vi "Get Command Line Arguments.vi"(8 "error in (no error)":errorcluster) -> (0 "error out":errorcluster, 2 "arguments":string[](array[string]), 3 "application name":string)   [LabVIEW 2020]
doc: "Returns the arguments passed from the command line when LabVIEW or a LabVIEW-built application launched. User-defined arguments start after two hyphens (--) surrounded by spaces in the command line.\n\nIf an argument contains double quotation marks (\"), this VI returns the argument without the quotation marks."
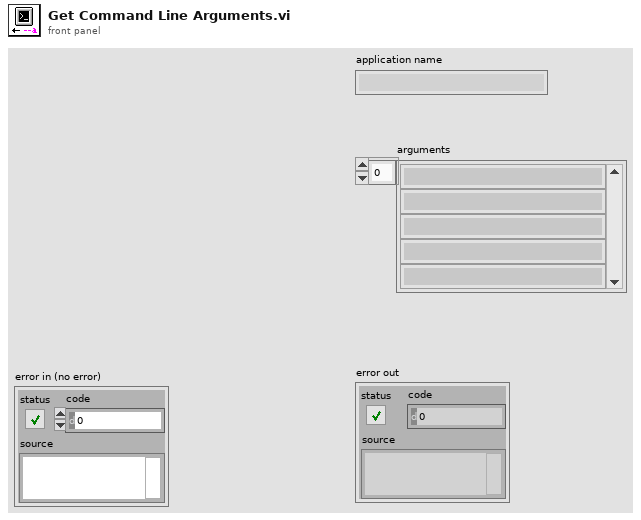
[diagram p1: front panel]
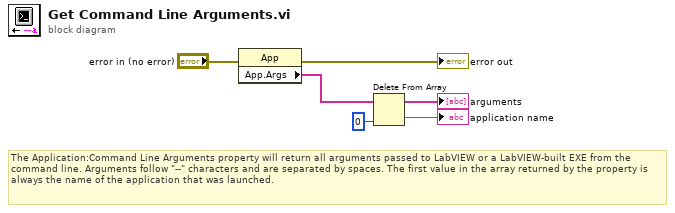
[diagram p0: block diagram]
diagram:
  # "The Application:Command Line Arguments property will return all arguments passed to LabVIEW or a LabVIEW-built EXE from the command line. Arguments follow \"--\" characters and are separated by spaces. The first value in the array returned by the property is always the name of the application that was launched."
  n1 = property class="App"(error in="error in (no error)") -> (error out=→"error out":errorcluster, "App.Args"=w4:string[])  [unwired: 1 in, 1 out]
  n2 = Delete From Array(array=w4, index=0) -> (deleted portion=→"application name":string, array with subset deleted=→"arguments":string[])  [unwired: 1 in]
